vi "salRegSubEvents.vi"(8 "error in (no error)":errorcluster, 11 "MiddlewareSALThisComponent in":refnum<class "MiddlewareSALThisComponent.lvclass">) -> (0 "error out":errorcluster, 3 "MiddlewareSALThisComponent out":refnum<class "MiddlewareSALThisComponent.lvclass">)   [LabVIEW 2016, in "MiddlewareSALThisComponent.lvclass"]
uses:
  MiddlewareSALThisComponent.lvclass
  SALCommunicatorDL/SALCommunicatorDL.lvclass
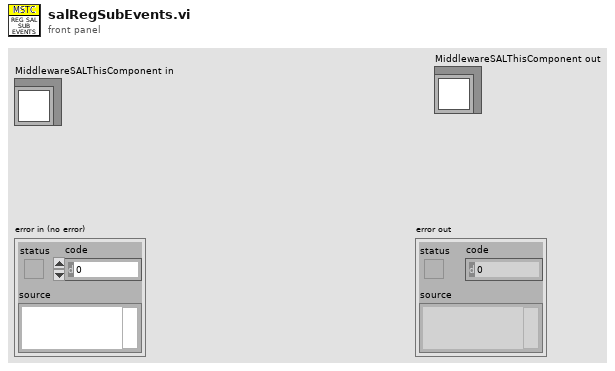
[diagram p1: front panel]
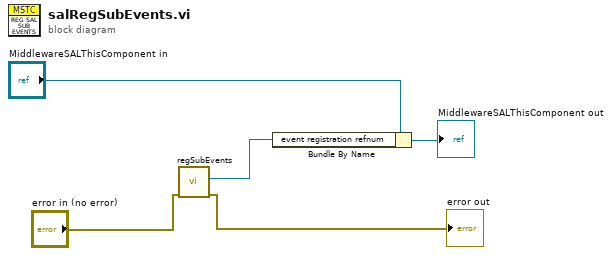
[diagram p0: block diagram]
diagram:
  n1 = call "regSubEvents.vi"("error in (no error)"="error in (no error)") -> ("error out"=→"error out":errorcluster, "Event Registration Refnum"=w4:refnum<event-registration>)  [unwired: 8 in, 1 out]
  n2 = Bundle By Name(cluster="MiddlewareSALThisComponent in", "event registration refnum"=w4) -> (→"MiddlewareSALThisComponent out":refnum<class "MiddlewareSALThisComponent.lvclass">)
